vi "VI Tree.vi"   [LabVIEW 2010, in "Agilent U2722.lvlib"]
doc: "This is the instrument driver for the Agilent U2722A and U2723A USB Modular Source Measure Unit. The VI Tree displays all the user-callable VIs of the instrument driver in an organized table."
uses:
  Agilent U2722.lvlib
  Configure/Configure Channel (Current).vi
  Data/Read Output (Single).vi
panel:
  # "(c) 2009 National Instruments.  ALL RIGHTS RESERVED."
  # "SEE DIAGRAM\nFOR VI TREE."
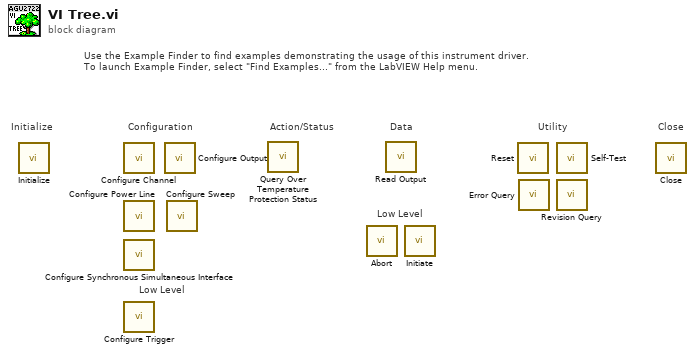
[diagram p0: block diagram]
diagram:
  # "Low Level"
  # "Low Level"
  # "Use the Example Finder to find examples demonstrating the usage of this instrument driver.\nTo launch Example Finder, select \"Find Examples...\" from the LabVIEW Help menu."
  # "Configuration"
  # "Utility"
  # "Data"
  # "Action/Status"
  # "Close"
  # "Initialize"
  n1 = call "Initialize.vi"() -> ()  [unwired: 10 in, 2 out]
  n2 = call-poly "Configure Channel.vi"() -> ()  [unwired: 10 in, 2 out]
  n3 = call "Configure Power Line.vi"() -> ()  [unwired: 10 in, 2 out]
  n4 = call "Configure Synchronous Simultaneous Interface.vi"() -> ()  [unwired: 10 in, 2 out]
  n5 = call "Configure Trigger.vi"() -> ()  [unwired: 10 in, 2 out]
  n6 = call "Configure Output.vi"() -> ()  [unwired: 10 in, 2 out]
  n7 = call "Configure Sweep.vi"() -> ()  [unwired: 10 in, 2 out]
  n8 = call "Query Over Temperature Protection Status.vi"() -> ()  [unwired: 9 in, 3 out]
  n9 = call "Abort.vi"() -> ()  [unwired: 10 in, 2 out]
  n10 = call-poly "Read Output.vi"() -> ()  [unwired: 8 in, 4 out]
  n11 = call "Initiate.vi"() -> ()  [unwired: 10 in, 2 out]
  n12 = call "Reset.vi"() -> ()  [unwired: 10 in, 2 out]
  n13 = call "Error Query.vi"() -> ()  [unwired: 8 in, 4 out]
  n14 = call "Self-Test.vi"() -> ()  [unwired: 8 in, 4 out]
  n15 = call "Revision Query.vi"() -> ()  [unwired: 8 in, 4 out]
  n16 = call "Close.vi"() -> ()  [unwired: 11 in, 1 out]
